vi "Location.vi"(10 "Port in":string, 11 "IP in":string) -> (2 "Longitude":string, 3 "Latitude":string)   [LabVIEW 2015]
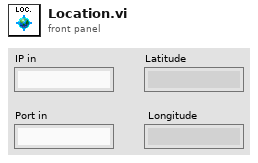
[diagram p1: front panel]
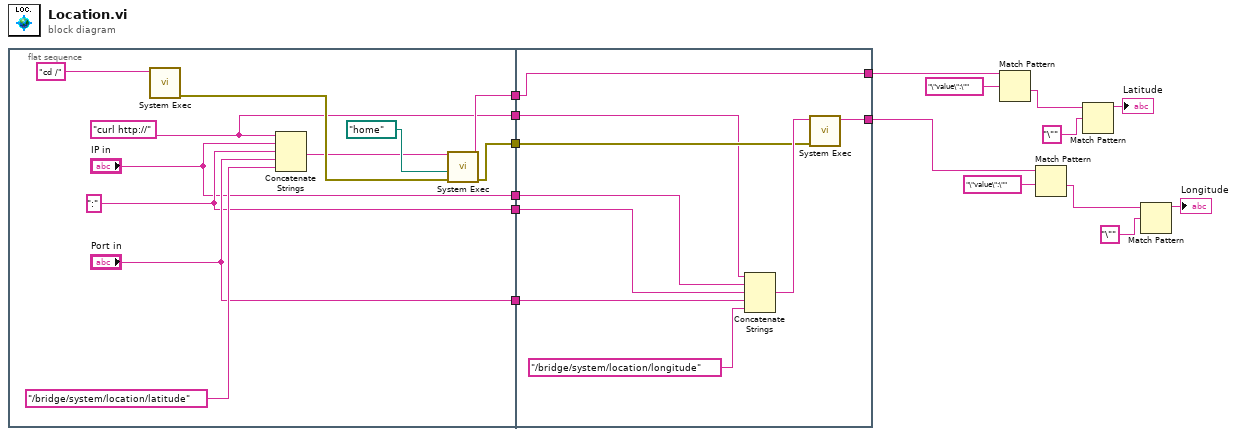
[diagram p0: block diagram]
diagram:
  n1 = flat-sequence {
    tunnel: [w22] -> w16
    tunnel: [w21] -> w15
    tunnel: ["Port in"] -> w14
    tunnel: [w19] -> w13
    tunnel: ["IP in"] -> w12
    tunnel: [w17] -> w11
    tunnel: [w34] -> w2
    tunnel: w16 -> [w33]
    tunnel: w15 -> [w32]
    tunnel: [w32] -> w1
    tunnel: w14 -> [w31]
    tunnel: w13 -> [w30]
    tunnel: w12 -> [w29]
    tunnel: w11 -> [w28]
    frame #0 {
      w19 = ":" ("string")
      w17 = "curl http://" ("string")
      n2 = call <vilib>:"System Exec.vi"("command line"="cd /") -> ("error out"=w25:errorcluster)  [unwired: 7 in, 3 out]
      n3 = Concatenate Strings(w17, "IP in", w19, "Port in", "/bridge/system/location/latitude" ("string")) -> (w23:string)
      n4 = call <vilib>:"System Exec.vi"("error in (no error)"=w25, "working directory"=path "/home", "command line"=w23) -> ("error out"=w22:errorcluster, "standard output"=w21:string)  [unwired: 5 in, 2 out]
    }
    frame #1 {
      n5 = Concatenate Strings(w28, w29, w30, w31, "/bridge/system/location/longitude" ("string")) -> (w36:string)
      n6 = call <vilib>:"System Exec.vi"("error in (no error)"=w33, "command line"=w36) -> ("standard output"=w34:string)  [unwired: 6 in, 3 out]
    }
  }
  n7 = Match Pattern(string=w1, regular expression="\"value\":\"") -> (after substring=w6:string)  [unwired: 1 in, 3 out]
  n8 = Match Pattern(string=w2, regular expression="\"value\":\"") -> (after substring=w10:string)  [unwired: 1 in, 3 out]
  n9 = Match Pattern(string=w6, regular expression="\"") -> (before substring=→"Latitude":string)  [unwired: 1 in, 3 out]
  n10 = Match Pattern(string=w10, regular expression="\"") -> (before substring=→"Longitude":string)  [unwired: 1 in, 3 out]
